vi "Integrity.vi"(8 "error in (no error)":errorcluster, 10 "user data":string="user ring data.ini", 11 "option lists":string="ring options.ini") -> (0 "error out":errorcluster)   [LabVIEW 2024]
doc: "Event-driven Queue State Machine (EDQSM) template in LabVIEW, designed to manage states and data via a queue. It includes three subVIs to create, enqueue, and dequeue states with attached data (using Variant for flexibility). The functional example features a simple interface with buttons that trigger events. The template is easily transformable into a traditional Queue State Machine (QSM) by removing the Wait state."
uses:
  controls/Data.ctl
  controls/ring data.ctl
  support/queue state & data (Array).vi
  <vilib>/Utility/error.llb/Error Cluster From Error Code.vi
  dependencies/read-write config ini string data.vi
  <vilib>/ErrorRing/Error Ring.xnode
  dependencies/read-write config ini.lvlib
  support/queue state & data.lvlib
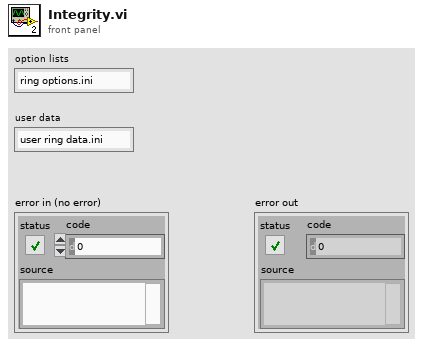
[diagram p1: front panel]
types:
  T1 = typedef "Data.ctl" = cluster{"Boolean":bool, "String":string, "Numeric":dbl, "option data":T2, "user data":T2}
  T2 = typedef "ring data.ctl" = cluster{"sectors":string[][], "key names":string[], "values":string[]}
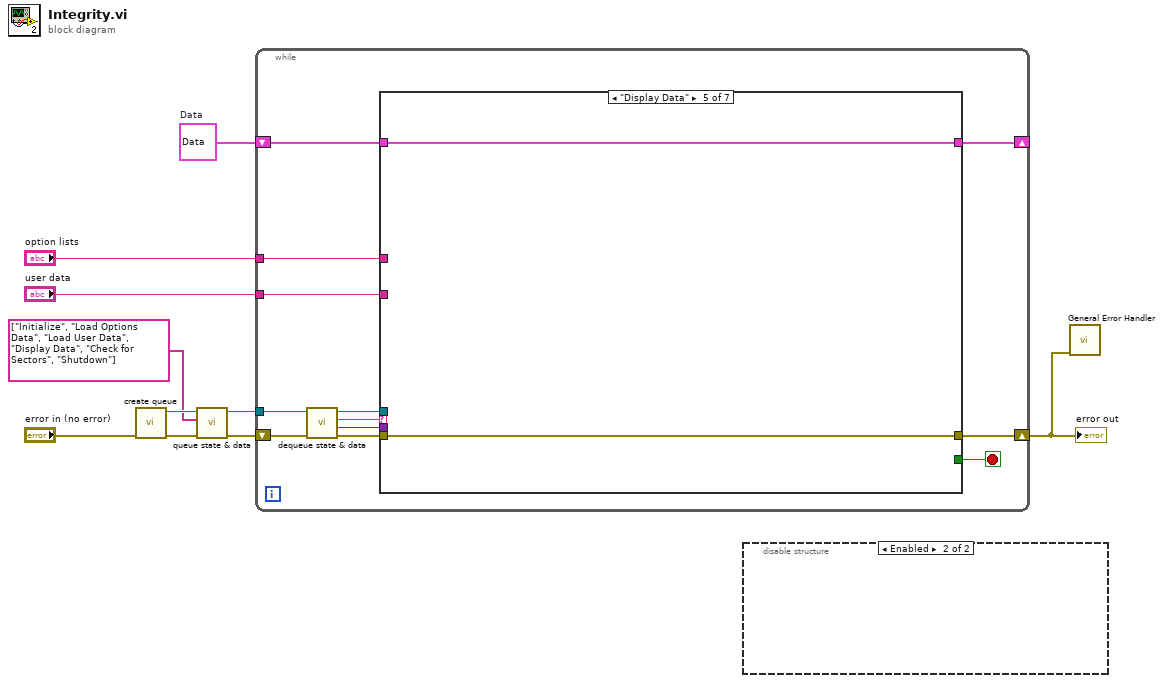
[diagram p0: block diagram]
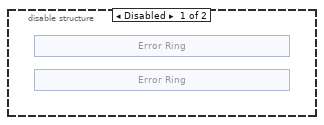
[diagram p2: hidden frame]
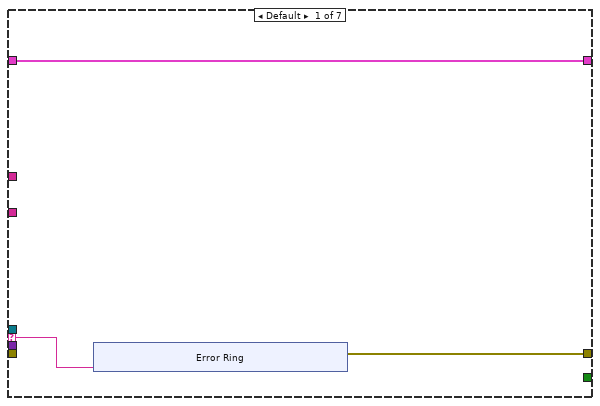
[diagram p3: hidden frame]
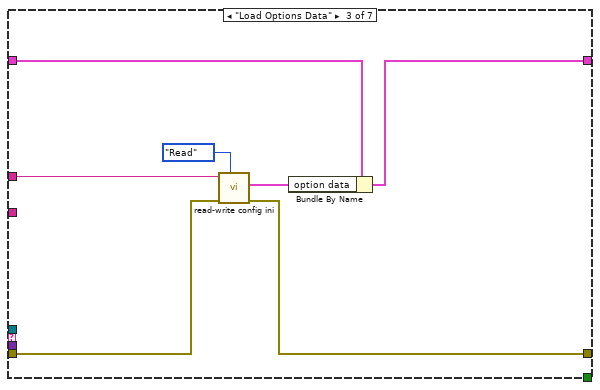
[diagram p5: hidden frame]
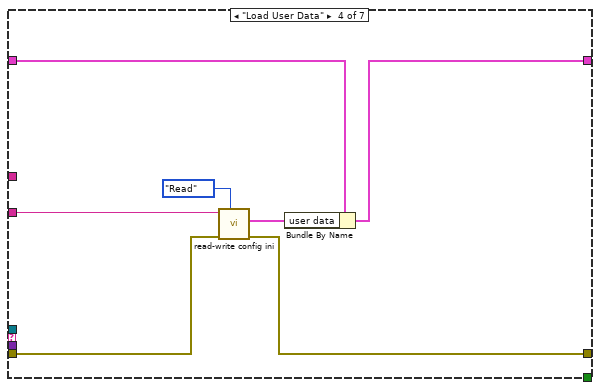
[diagram p6: hidden frame]
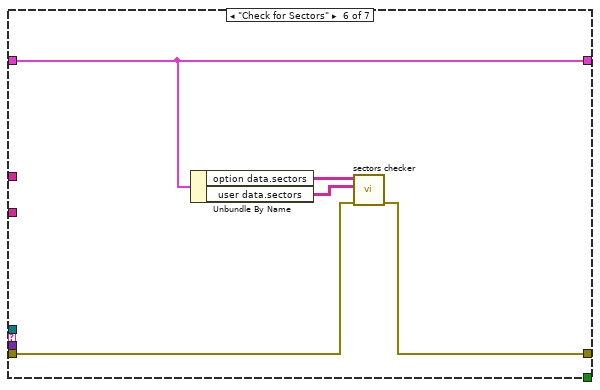
[diagram p7: hidden frame]
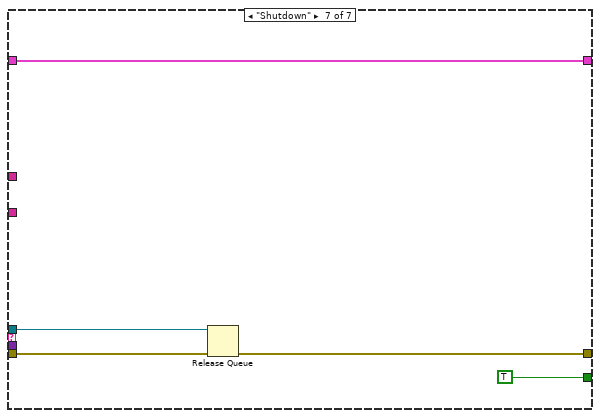
[diagram p8: hidden frame]
diagram:
  w6 = T1 {"Boolean"=FALSE, "String"="", "Numeric"=0.0, "option data"={"sectors"=[], "key names"=[], "values"=[]}, "user data"={"sectors"=[], "key names"=[], "values"=[]}}  # Data
  n1 = call "create queue.vi"("error in (no error)"="error in (no error)") -> ("error out"=w8:errorcluster, "queue out"=w10:refnum<queue>)  [unwired: 9 in]
  n2 = call-poly "queue state & data.vi"("error in (no error)"=w8, "State Array"=string[] ["Initialize", "Load Options Data", "Load User Data", "Display Data", "Check for Sectors", "Shutdown"], "queue in"=w10) -> ("error out"=w9:errorcluster, "queue out"=w7:refnum<queue>)  [unwired: 7 in]
  n3 = while {
    shift-right: [w22] -> w1
    shift-left: w9 -> [w17]
    tunnel: w7 -> [w15]
    shift-right: [w13] -> _
    shift-left: w6 -> [w14]
    tunnel: "user data" -> [w12]
    tunnel: "option lists" -> [w11]
    stop <- w21 stop-if-true
    n4 = call "dequeue state & data.vi"("error in (no error)"=w17, "queue in"=w15) -> ("error out"=w20:errorcluster, "State Data"=w18:variant, "State"=w19:string, "queue out"=w16:refnum<queue>)  [unwired: 6 in]
    n5 = case shown="\"Display Data\"" w19 {
      selector: w19 -> [w24 _ _ _ _ _ _]
      tunnel: w20 -> [_ w34 w39 w47 w49 w52 w59]
      tunnel: [w25 w34 w38 w46 w49 w51 w57] -> w22
      tunnel: [_ _ _ _ _ _ TRUE] -> w21
      tunnel: w16 -> [_ _ _ _ _ _ w58]
      tunnel: w18 -> [_ _ _ _ _ _ _]
      tunnel: w14 -> [w23 w33 w37 w45 w50 w55 w56]
      tunnel: [w23 w33 w35 w43 w50 w55 w56] -> w13
      tunnel: w12 -> [_ _ _ w42 _ _ _]
      tunnel: w11 -> [_ _ w40 _ _ _ _]
      frame Default {
        n6 = xnode "Error Ring"("parameter 0"=w24) -> ("error out"=w25:errorcluster)
      }
      frame "Initialize" {
      }
      frame "Load Options Data" {
        n7 = call-poly "read-write config ini.vi"("Function"=enum16{"Read", "Write"}."Read", "error in (no error)"=w39, "file name"=w40) -> ("error out"=w38:errorcluster, "user data out"=w36:T2)  [unwired: 7 in]
        n8 = Bundle By Name(cluster=w37, "option data"=w36) -> (w35:T1)
      }
      frame "Load User Data" {
        n9 = call-poly "read-write config ini.vi"("Function"=enum16{"Read", "Write"}."Read", "error in (no error)"=w47, "file name"=w42) -> ("error out"=w46:errorcluster, "user data out"=w44:T2)  [unwired: 7 in]
        n10 = Bundle By Name(cluster=w45, "user data"=w44) -> (w43:T1)
      }
      frame "Display Data" {
      }
      frame "Check for Sectors" {
        n11 = Unbundle By Name(w55) -> ("option data.sectors"=w54:string[][], "user data.sectors"=w53:string[][])
        n12 = call "sectors checker.vi"("error in (no error)"=w52, "array2"=w53, "array1"=w54) -> ("error out"=w51:errorcluster)  [unwired: 8 in]
      }
      frame "Shutdown" {
        n13 = Release Queue(queue=w58, error in (no error)=w59) -> (error out=w57:errorcluster)  [unwired: 1 in, 2 out]
      }
    }
  }
  "error out" <- w1
  n14 = disable-structure shown="Enabled" {
    frame Disabled {
      n15 = xnode "Error Ring"() -> ()  [unwired: 1 out]
      n16 = xnode "Error Ring"() -> ()  [unwired: 1 out]
    }
    frame Enabled {
    }
  }
  n17 = call <vilib>:"General Error Handler.vi"("error in (no error)"=w1) -> ()  [unwired: 10 in, 5 out]
